vi "DSF.Shared.Timing.Get Priority.vi"(11 "Timing in":refnum<class "DSF.Shared.Timing.lvclass">) -> (2 "Priority":u64, 3 "Timing out":refnum<class "DSF.Shared.Timing.lvclass">)   [LabVIEW 2017, in "DSF.Shared.lvlib" / "DSF.Shared.Timing.lvclass"]
uses:
  DSF.Shared.Timing.lvclass
  DSF.Shared.Timing.lvclass/DSF.Shared.Timing.ctl
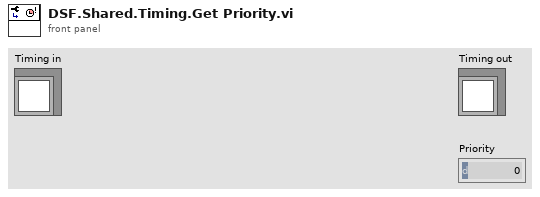
[diagram p1: front panel]
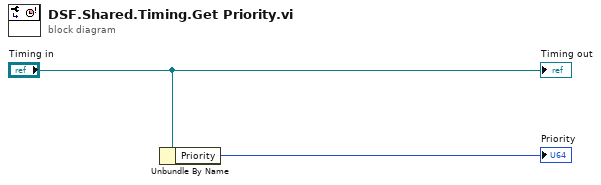
[diagram p0: block diagram]
diagram:
  n1 = Unbundle By Name("Timing in") -> ("Priority"=→"Priority":u64)
  "Timing out" <- "Timing in"
